vi "KepcoDCPwr Software Timed Ramp Example.vi"(0 "VISA resource name":refnum<visa-resource-name>="GPIB0::6::INSTR", 1 "Boolean":bool=TRUE, 7 "Model In":string, 11 "error in (no error)":errorcluster) -> (8 "End voltage":dbl, 15 "error out":errorcluster)   [LabVIEW 2013]
panel:
  in  "Exit":bool
  in  "Start":bool
  in  "Ramp Direction":bool=TRUE
  out "Voltage vs Time":cluster{dbl[], dbl[]}(graph)
  in  "Readback Current":bool
  in  "Readback Voltage":bool
  in  "Voltage Increment":dbl=1.0 format="%.2f"
  in  "Dwell (ms)":u32=50 min=100 max=5000 step=1
  in  "End (Volts)":dbl=10.0 format="%.2f"
  in  "Start (Volts)":dbl format="%.2f"
  in  "# of Cycles":i32
  in  "Repeat":bool=TRUE
  in  "Disable @ End":bool
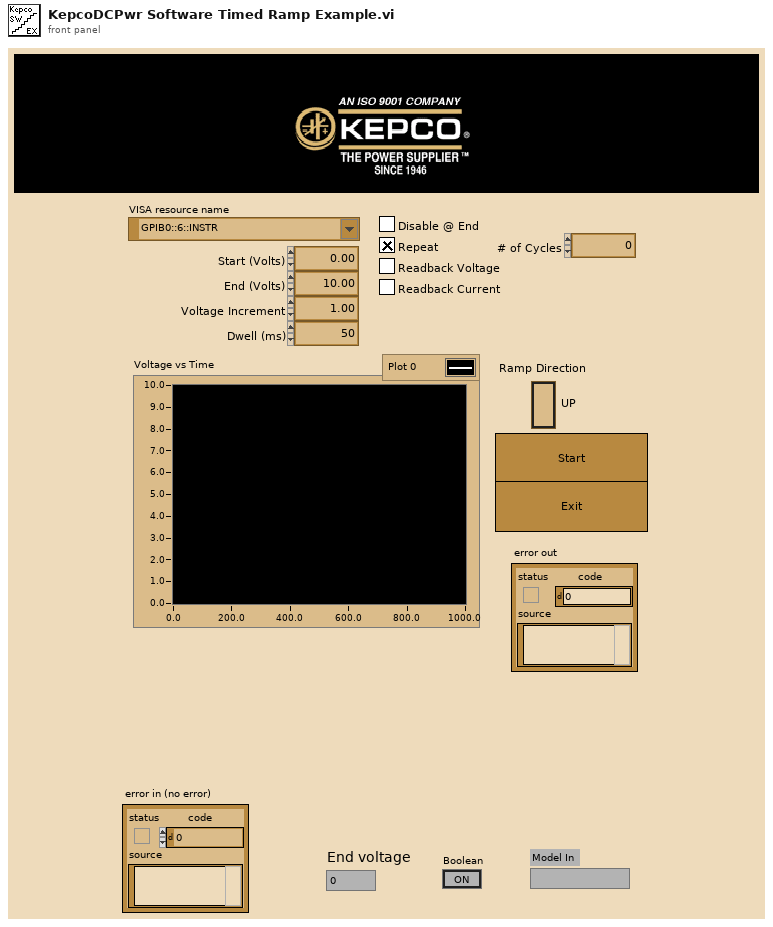
[diagram p1: front panel]
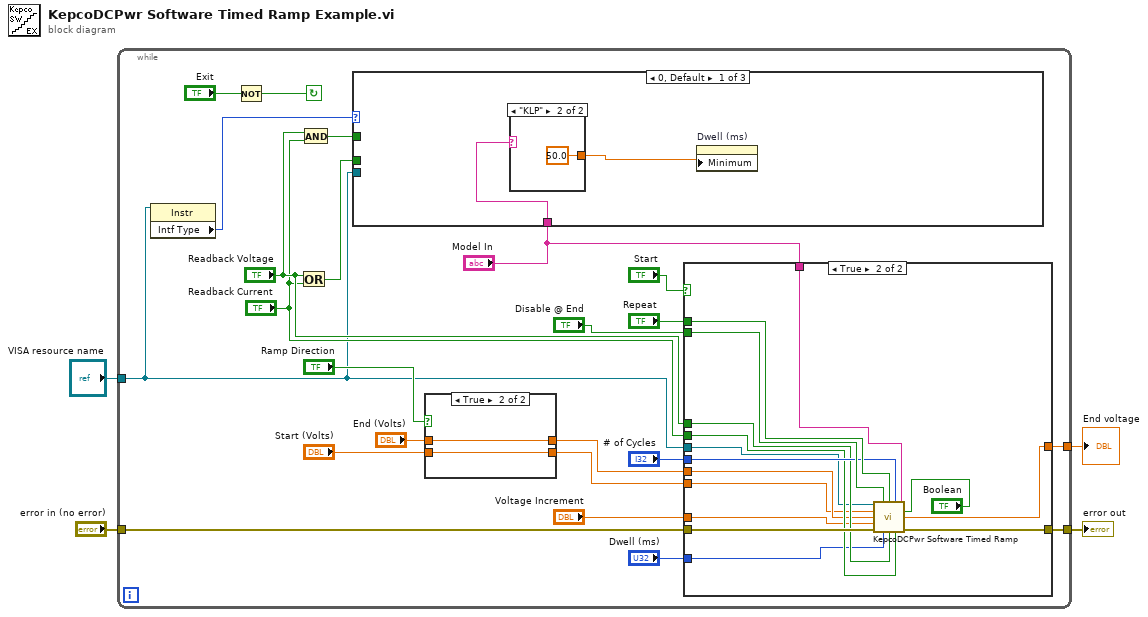
[diagram p0: block diagram]
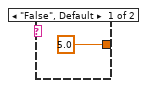
[diagram p2: hidden frame]
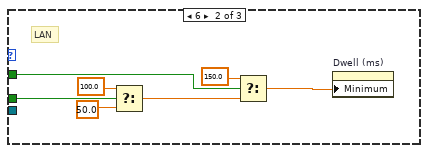
[diagram p3: hidden frame]
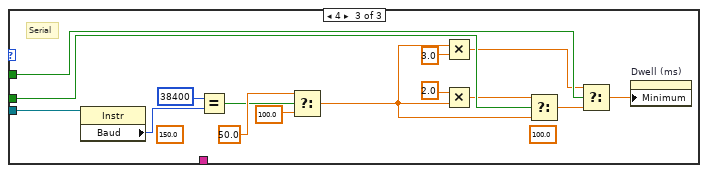
[diagram p4: hidden frame]
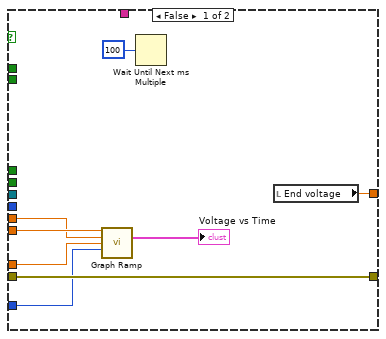
[diagram p5: hidden frame]
diagram:
  n1 = while {
    tunnel: "VISA resource name" -> [w6]
    tunnel: [w26] -> w3
    tunnel: "error in (no error)" -> [w27]
    tunnel: [w12] -> w1
    stop <- w16 continue-if-true
    n2 = property class="Instr"(reference=w6) -> ("Intf Type"=w11:u16)  [unwired: 1 in, 2 out]
    n3 = Not(x="Exit") -> (.not. x?=w16:bool)
    n4 = Or(x="Readback Voltage", y="Readback Current") -> (x .or. y?=w7:bool)
    n5 = And(x="Readback Voltage", y="Readback Current") -> (x .and. y?=w8:bool)
    n6 = case shown="0, Default" w11 {
      tunnel: w7 -> [_ w34 w50]
      tunnel: w8 -> [_ w36 w51]
      tunnel: w6 -> [_ _ w49]
      tunnel: "Model In" -> [w29 _ _]
      frame 0, Default {
        n7 = case shown="\"KLP\"" w29 {
          tunnel: [5.0 ("Data Entry Limits:Minimum") 50.0 ("Data Entry Limits:Minimum")] -> w28
          frame "False", Default {
          }
          frame "KLP" {
          }
        }
        n8 = property on="Dwell (ms)" class="DigNum (strict)"("Minimum"=w28) -> ()  [unwired: 2 in, 2 out]
      }
      frame 6 {
        # "LAN"
        n9 = Select(t=100.0, s=w34, f=50.0) -> (s? t:f=w37:dbl)
        n10 = Select(t=150.0, s=w36, f=w37) -> (s? t:f=w38:dbl)
        n11 = property on="Dwell (ms)" class="DigNum (strict)"("Minimum"=w38) -> ()  [unwired: 2 in, 2 out]
      }
      frame 4 {
        (unwired) 100.0 ("t")
        (unwired) 150.0 ("t")
        # "Serial"
        n12 = property class="Instr"(reference=w49) -> ("Baud"=w43:u32)  [unwired: 1 in, 2 out]
        n13 = Equal?(x=u32 38400, y=w43) -> (x = y?=w42:bool)
        n14 = Select(t=50.0 ("f"), s=w42, f=100.0) -> (s? t:f=w39:dbl)
        n15 = Multiply(x=w39, y=3.0) -> (x*y=w46:dbl)
        n16 = Multiply(x=2.0, y=w39) -> (x*y=w45:dbl)
        n17 = Select(t=w45, s=w50, f=w39) -> (s? t:f=w52:dbl)
        n18 = Select(t=w46, s=w51, f=w52) -> (s? t:f=w53:dbl)
        n19 = property on="Dwell (ms)" class="DigNum (strict)"("Minimum"=w53) -> ()  [unwired: 2 in, 2 out]
      }
    }
    n20 = case shown="True" "Ramp Direction" {
      tunnel: "End (Volts)" -> [w78 w79]
      tunnel: "Start (Volts)" -> [w77 w80]
      tunnel: [w78 w80] -> w18
      tunnel: [w77 w79] -> w17
      frame False {
      }
      frame True {
      }
    }
    n21 = case shown="True" "Start" {
      tunnel: w27 -> [w61 w76]
      tunnel: [w61 w75] -> w26
      tunnel: "Dwell (ms)" -> [w56 w69]
      tunnel: "Voltage Increment" -> [w57 w68]
      tunnel: "Readback Current" -> [_ w71]
      tunnel: "Readback Voltage" -> [_ w70]
      tunnel: "Disable @ End" -> [_ w74]
      tunnel: "Repeat" -> [_ w73]
      tunnel: "# of Cycles" -> [_ w72]
      tunnel: w18 -> [w59 w66]
      tunnel: w17 -> [w58 w67]
      tunnel: w6 -> [_ w65]
      tunnel: [w54 w63] -> w12
      tunnel: "Model In" -> [_ w62]
      frame False {
        n22 = call "Graph Ramp.vi"("Start (Volts)"=w59, "End (volts)"=w58, "Voltage Increment"=w57, "Dwell (sec)"=w56) -> ("Voltage vs Time"=→"Voltage vs Time":cluster{dbl[], dbl[]})  [unwired: 11 out]
        n23 = Wait Until Next ms Multiple(millisecond multiple=u32 100) -> ()  [unwired: 1 out]
        n24 = local read "End voltage"() -> (w54:dbl)
      }
      frame True {
        n25 = call "KepcoDCPwr Software Timed Ramp.vi"("VISA resource name"=w65, "Disable @ End"=w74, "Repeat"=w73, "# of Cycles"=w72, "Model In"=w62, "Start (Volts)"=w66, "Boolean"="Boolean", "End (Volts)"=w67, "Voltage Increment"=w68, "error in (no error)"=w76, "Dwell (ms)"=w69, "Readback Voltage"=w70, "Readback Current"=w71) -> ("End voltage"=w63:dbl, "error out"=w75:errorcluster)  [unwired: 1 out]
      }
    }
  }
  "error out" <- w3
  "End voltage" <- w1
